vi "documentFactory (by File Extension).vi"(8 "error in (no error)":errorcluster, 11 "File Path":path) -> (0 "error out":errorcluster, 1 "dup file":path, 3 "npoiDocument out":refnum<class "npoiDocument.lvclass">)   [LabVIEW 2017, in "Document API.lvlib" / "Document API.lvclass"]
uses:
  Document API.lvclass
  NPOI_Document/npoiDocument/npoiDocument.lvclass
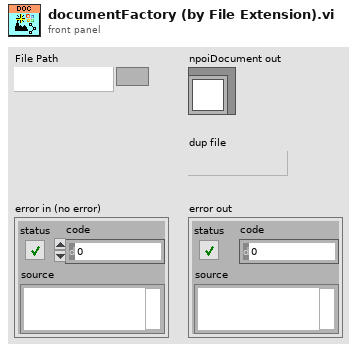
[diagram p1: front panel]
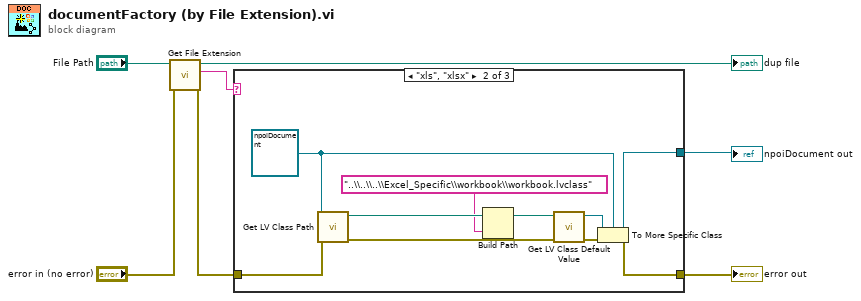
[diagram p0: block diagram]
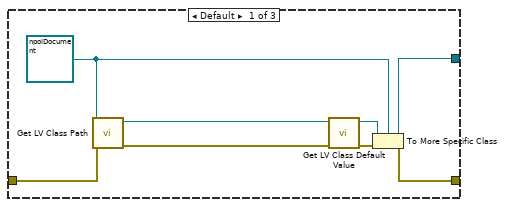
[diagram p2: hidden frame]
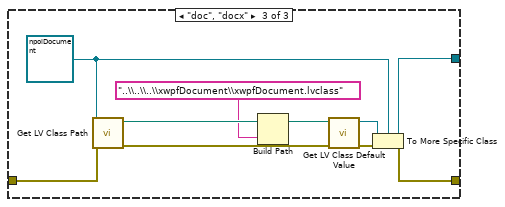
[diagram p3: hidden frame]
diagram:
  n1 = call <vilib>:"Get File Extension.vi"("error in (no error)"="error in (no error)", "file"="File Path") -> ("error out"=w1:errorcluster, "lowercase file extension"=w3:string, "dup file"=→"dup file":path)  [unwired: 5 in, 2 out]
  n2 = case shown="\"xls\", \"xlsx\"" w3 {
    tunnel: [w15 w25 w35] -> w5
    tunnel: w1 -> [w14 w24 w34]
    tunnel: [w13 w23 w33] -> w6
    frame Default {
      w12 = refnum<class "npoiDocument.lvclass"> refnum ("NPOI_Document.lvlib:npoiDocument.lvclass")
      n3 = call <vilib>:"Get LV Class Path.vi"("error in (no error)"=w14, "object"=w12) -> ("error out"=w11:errorcluster, "class path"=w10:path)  [unwired: 8 in]
      n4 = call <vilib>:"Get LV Class Default Value.vi"("error in (no error)"=w11, "class path"=w10) -> ("error out"=w9:errorcluster, "object"=w8:refnum<class>)  [unwired: 8 in]
      n5 = To More Specific Class(target class=w12, reference=w8, error in=w9) -> (specific class reference=w15:refnum<class "npoiDocument.lvclass">, error out=w13:errorcluster)
    }
    frame "xls", "xlsx" {
      w22 = refnum<class "npoiDocument.lvclass"> refnum ("NPOI_Document.lvlib:npoiDocument.lvclass")
      n6 = call <vilib>:"Get LV Class Path.vi"("error in (no error)"=w24, "object"=w22) -> ("error out"=w21:errorcluster, "class path"=w20:path)  [unwired: 8 in]
      n7 = Build Path(base path=w20, name or relative path="..\\..\\..\\Excel_Specific\\workbook\\workbook.lvclass") -> (appended path=w17:path)
      n8 = call <vilib>:"Get LV Class Default Value.vi"("error in (no error)"=w21, "class path"=w17) -> ("error out"=w19:errorcluster, "object"=w18:refnum<class>)  [unwired: 8 in]
      n9 = To More Specific Class(target class=w22, reference=w18, error in=w19) -> (specific class reference=w25:refnum<class "npoiDocument.lvclass">, error out=w23:errorcluster)
    }
    frame "doc", "docx" {
      w32 = refnum<class "npoiDocument.lvclass"> refnum ("NPOI_Document.lvlib:npoiDocument.lvclass")
      n10 = call <vilib>:"Get LV Class Path.vi"("error in (no error)"=w34, "object"=w32) -> ("error out"=w31:errorcluster, "class path"=w30:path)  [unwired: 8 in]
      n11 = Build Path(base path=w30, name or relative path="..\\..\\..\\xwpfDocument\\xwpfDocument.lvclass") -> (appended path=w27:path)
      n12 = call <vilib>:"Get LV Class Default Value.vi"("error in (no error)"=w31, "class path"=w27) -> ("error out"=w29:errorcluster, "object"=w28:refnum<class>)  [unwired: 8 in]
      n13 = To More Specific Class(target class=w32, reference=w28, error in=w29) -> (specific class reference=w35:refnum<class "npoiDocument.lvclass">, error out=w33:errorcluster)
    }
  }
  "error out" <- w6
  "npoiDocument out" <- w5
